vi "Costo Update.vi"(8 "error in (no error)":errorcluster, 10 "Costo":dbl, 11 "UI in":refnum<class "UI.lvclass">) -> (0 "error out":errorcluster, 3 "UI out":refnum<class "UI.lvclass">)   [LabVIEW 2021, in "UI.lvlib" / "UI.lvclass"]
uses:
  UI.lvclass
  UI.lvclass/UI.ctl
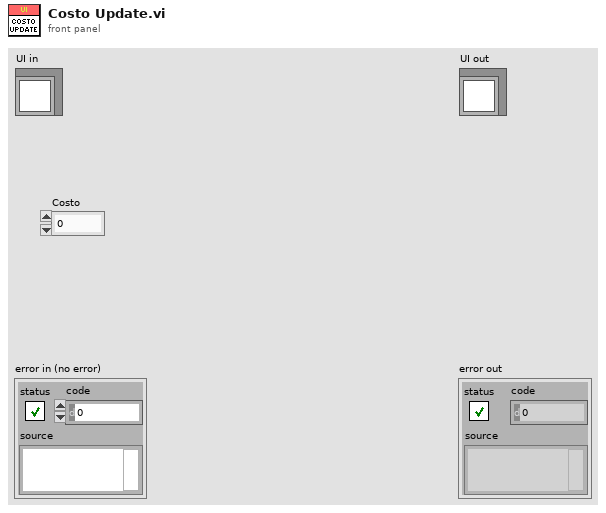
[diagram p1: front panel]
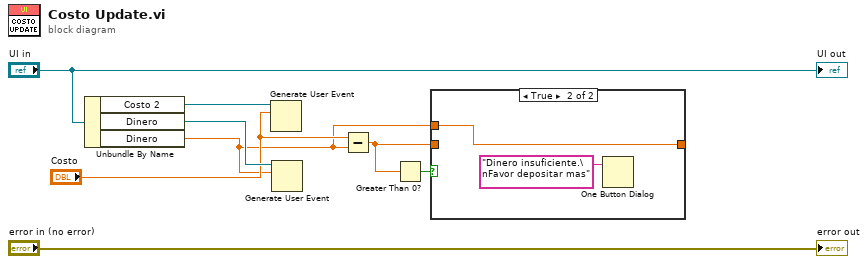
[diagram p0: block diagram]
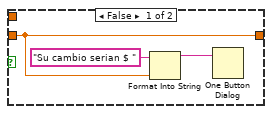
[diagram p2: hidden frame]
diagram:
  n1 = Unbundle By Name("UI in") -> ("Costo 2"=w6:refnum<user-event>, "Dinero"=w5:refnum<user-event>, "Dinero"=w1:dbl)
  n2 = Generate User Event(user event=w6, event data cluster="Costo") -> ()  [unwired: 2 in, 2 out]
  n3 = Generate User Event(user event=w5, event data cluster=w1) -> ()  [unwired: 2 in, 2 out]
  n4 = Subtract(x="Costo", y=w1) -> (x-y=w2:dbl)
  n5 = Greater Than 0?(x=w2) -> (x > 0?=w3:bool)
  n6 = case shown="True" w3 {
    tunnel: w2 -> [w10 _]
    tunnel: [w10 w12] -> _
    tunnel: w1 -> [_ w12]
    frame False {
      n7 = Format Into String(initial string="Su cambio serian $ ", w10) -> (resulting string=w9:string)  [unwired: 2 in, 1 out]
      n8 = One Button Dialog(message=w9) -> ()  [unwired: 1 in, 1 out]
    }
    frame True {
      n9 = One Button Dialog(message="Dinero insuficiente.\nFavor depositar mas") -> ()  [unwired: 1 in, 1 out]
    }
  }
  "error out" <- "error in (no error)"
  "UI out" <- "UI in"
